vi "MainStateMachine.vi"() -> ()   [LabVIEW 2018]
uses:
  <vilib>/platform/TimedLoop/XDataNode/XDataNode.xnode
  <vilib>/Platform/TimedLoop/XDataNode/nitl_modes.ctl
  <vilib>/Platform/TimedLoop/XDataNode/XDNodeRunTimeDep.lvlib
  <vilib>/Platform/TimedLoop/XDataNode/wakeup.ctl
  <vilib>/Platform/TimedLoop/XDataNode/timing_clust.ctl
  Type_Def_ControlState.ctl
  <vilib>/Platform/TimedLoop/XDataNode/loadnilvce.vi
  Type_Def Actuator Controls.ctl
  C:/Users/eric/Documents/LabViewBuilds/Testing/FaultPractice/Type_Def SensorData.ctl
  2019_CompetitionCode-master/2019_CompetitionCode-master/Master/DAQ/TypeDef_cRIOData.ctl
panel:
  in  "error constant":errorcluster
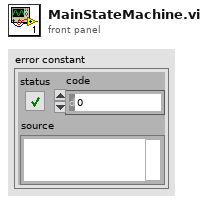
[diagram p1: front panel]
types:
  T1 = typedef "Type_Def Actuator Controls.ctl" = cluster{"Reverse ":bool, "Forward":bool, "Low Side":bool, "Precharge":bool, "High Side":bool, "Digital Out 5":bool, "Digital Out 6":bool, "Digital Out 7 ":bool, "24 Power":bool, "Tank Valve ":bool, "Brake Valve":bool, "Pump":bool, "Digital Out 1 ":bool, "Digital Out 2":bool, "Digital Out 3":bool, "Digital Out 4 ":bool}
  T2 = typedef "Type_Def_ControlState.ctl" = enum16{"Blank", "Systems Check", "Idle", "Ready", "Pushing", "CrawlingPrecharge", "Braking", "Fault", "Boot Up", "Unpowered", "Crawling", "Shutdown", "Service Push", "Service Wait", "Vent", "Precharge", "Cooldown"}
  T3 = typedef "Type_Def SensorData.ctl" = cluster{"cRIO Data":T4}
  T4 = typedef "TypeDef_cRIOData.ctl" = cluster{"Time (ms)":dbl, "24V Battery (V)":dbl, "LowV Current (A)":dbl, "Fiducial Sensor (V)":dbl, "PV Pressure (psig)":dbl, "Flow Sensor (V)":dbl, "Temp Fairing (F)":dbl, "Temp Reservoir (F)":dbl, "HallEffect Right (in)":dbl, "HallEffect Left (in)":dbl, "PT Tank (psig)":dbl, "PT Clamp Right (psig)":dbl, "PT Clamp Left (psig)":dbl, "PT Brake (psig)":dbl, "PT Cooling (psig)":dbl, "Displacement (ft)":dbl, "Velocity (ft/s)":dbl}
  T5 = cluster{"cRIO Data":cluster{"Time (ms)":dbl, "24V Battery (V)":dbl, "LowV Current (A)":dbl, "Fiducial Sensor (V)":dbl, "PV Pressure (psig)":dbl, "Flow Sensor (V)":dbl, "Temp Fairing (F)":dbl, "Temp Reservoir (F)":dbl, "HallEffect Right (in)":dbl, "HallEffect Left (in)":dbl, "PT Tank (psig)":dbl, "PT Clamp Right (psig)":dbl, "PT Clamp Left (psig)":dbl, "PT Brake (psig)":dbl, "PT Cooling (psig)":dbl, "Displacement (ft)":dbl, "Velocity (ft/s)":dbl}}
  T6 = typedef "Type_Def ClusterSensor.ctl" = cluster{"Sensor Data":dbl, "Max":dbl, "Min":dbl, "Previous Data":dbl, "#same":dbl}
  T7 = typedef "XDNodeRunTimeDep.lvlib/timing_clust.ctl" = cluster{"Expected End [f-1]":u64, "Actual End [f-1]":u64, "Finished Late? [f-1]":bool, "Expected End [i-1]":u64, "Actual End [i-1]":u64, "Finished Late? [i-1]":bool, "Expected Start [i]":u64, "Actual Start [i]":u64, "Expected Start [f]":u64, "Actual Start [f]":u64, "Source Name":string, "Structure Name":string, "Period":i64, "Deadline":i64, "Offset":i64, "Start":i64, "Priority":i32, "Timeout":i32, "Mode":T8, "Wakeup Reason":T9, "Error":errorcluster, "Source Type":string, "Secondary Source Type":string, "Global End Time":u64, "Global Start Time":u64, "Frame Duration":u64, "Iteration Duration":u64, "Assigned CPU":i32, "I/O Scan Engine Mode":u32}
  T8 = typedef "XDNodeRunTimeDep.lvlib/nitl_modes.ctl" = enum32{"No Change", "Process missed periods, maintain original phase", "Discard missed periods, maintain original phase", "Process missed periods, ignore original phase", "Discard missed periods, ignore original phase"}
  T9 = typedef "XDNodeRunTimeDep.lvlib/wakeup.ctl" = enum32{"Normal", "Aborted", "Asynchronous wakeup", "Timing source error", "Timed loop error", "Timeout"}
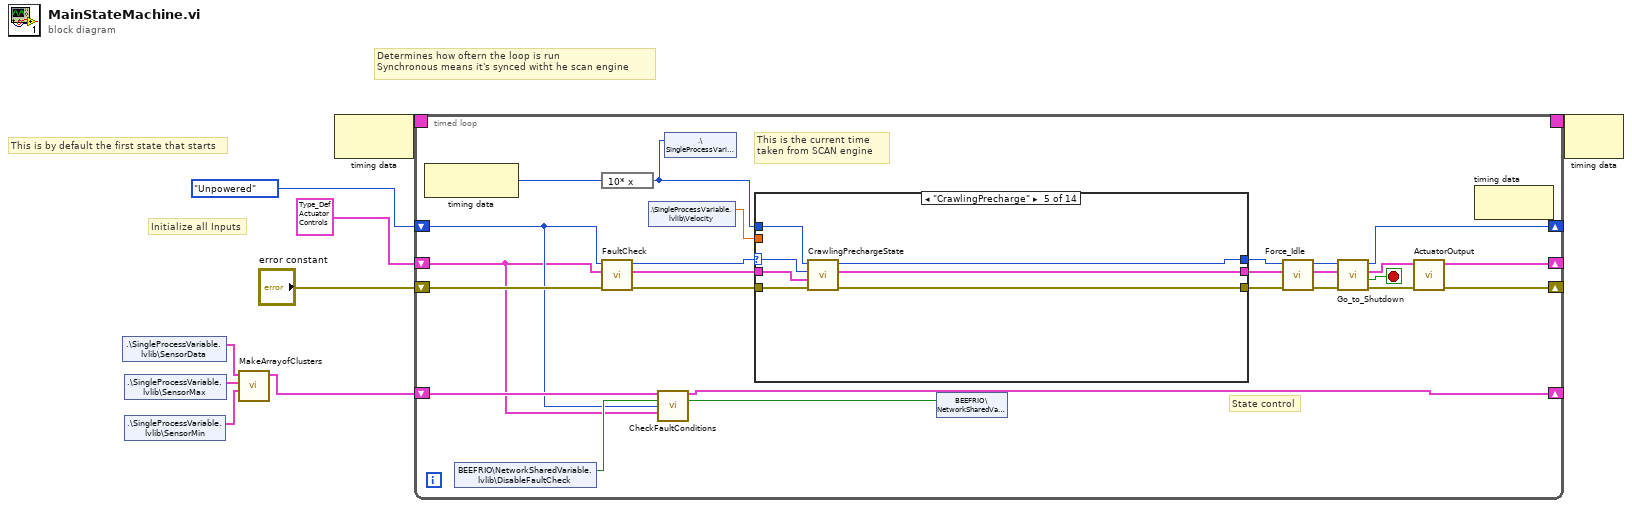
[diagram p0: block diagram]
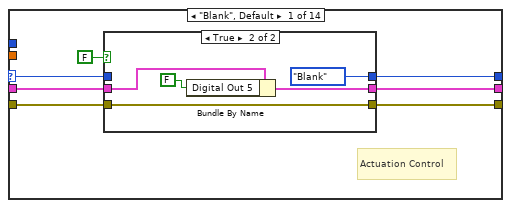
[diagram p2: hidden frame]
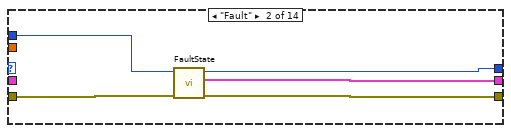
[diagram p4: hidden frame]
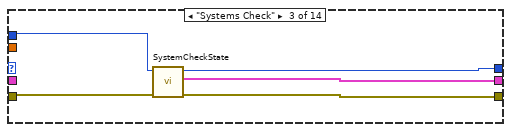
[diagram p5: hidden frame]
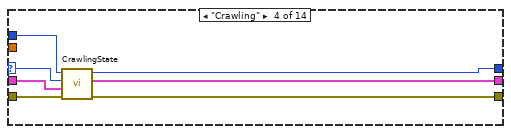
[diagram p6: hidden frame]
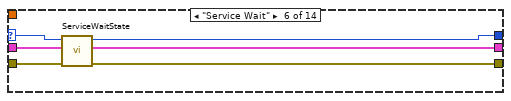
[diagram p7: hidden frame]
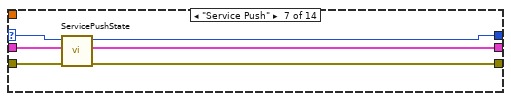
[diagram p8: hidden frame]
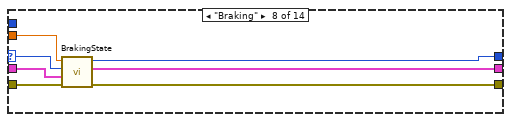
[diagram p9: hidden frame]
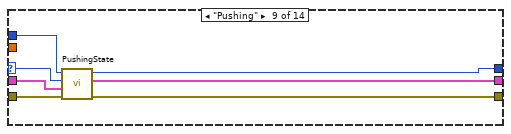
[diagram p10: hidden frame]
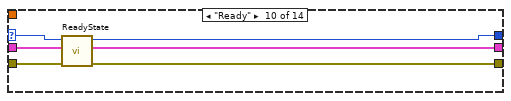
[diagram p11: hidden frame]
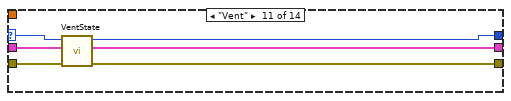
[diagram p12: hidden frame]
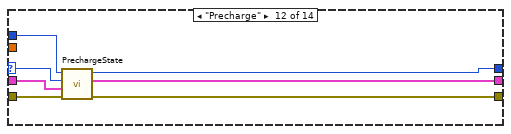
[diagram p13: hidden frame]
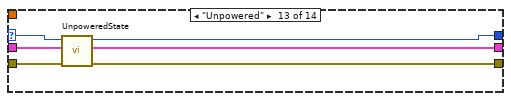
[diagram p14: hidden frame]
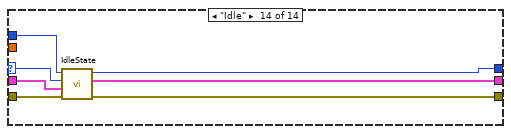
[diagram p15: hidden frame]
diagram:
  # "Determines how oftern the loop is run \nSynchronous means it's synced witht he scan engine"
  # "Initialize all Inputs"
  # "This is by default the first state that starts"
  n1 = shared-variable ".\\SingleProcessVariable.lvlib\\SensorData"() -> (w4:T3)  [unwired: 1 in, 1 out]
  n2 = shared-variable ".\\SingleProcessVariable.lvlib\\SensorMax"() -> (w3:T5)  [unwired: 1 in, 1 out]
  n3 = shared-variable ".\\SingleProcessVariable.lvlib\\SensorMin"() -> (w2:T3)  [unwired: 1 in, 1 out]
  n4 = call "MakeArrayofClusters.vi"(9:"SensorMax"=w2, 10:"SensorMax"=w3, "SensorData"=w4) -> ("Array"=w1:cluster{"SensorCluster":T6}[])  [unwired: 8 in]
  n5 = node-c288() -> (w9:T7)  [unwired: 1 in]
  n6 = timed-loop {
    timing: w9 -> [_]
    timing-out: [_] -> w8
    shift-right: [w33] -> _
    shift-left: Type_Def_ControlState."Unpowered" -> [w12]
    shift-right: [w21] -> _
    shift-left: T1 {"Reverse "=FALSE, "Forward"=FALSE, "Low Side"=FALSE, "Precharge"=FALSE, "High Side"=FALSE, "Digital Out 5"=FALSE, "Digital Out 6"=FALSE, "Digital Out 7 "=FALSE, "24 Power"=FALSE, "Tank Valve "=FALSE, "Brake Valve"=FALSE, "Pump"=FALSE, "Digital Out 1 "=FALSE, "Digital Out 2"=FALSE, "Digital Out 3"=FALSE, "Digital Out 4 "=FALSE} -> [w10]
    shift-right: [w20] -> _
    shift-left: "error constant" -> [w34]
    shift-right: [w15] -> _
    shift-left: w1 -> [w14]
    stop <- w24 stop-if-true
    # "This is the current time \ntaken from SCAN engine"
    # "State control"
    n7 = node-c288() -> (w23:i64)  [unwired: 1 in]
    n8 = shared-variable "BEEFRIO\\NetworkSharedVariable.lvlib\\DisableFaultCheck"() -> (w13:bool)  [unwired: 1 in, 1 out]
    n9 = expression code="10* x"(w23) -> (w22:i64)
    n10 = call "FaultCheck.vi"("error in (no error)"=w34, "Cluster in"=w10, "Enum in"=w12) -> ("error out"=w16:errorcluster, "Cluster out"=w17:T1, "Enum out"=w18:T2)  [unwired: 6 in]
    n11 = shared-variable ".\\SingleProcessVariable.lvlib\\Velocity"() -> (w19:dbl)  [unwired: 1 in, 1 out]
    n12 = call "CheckFaultConditions.vi"(0:w14, "DisableFaultCheck"=w13, "ControlState"=w12, "Cluster"=w10) -> ("Array out"=w15:cluster{"SensorCluster":T6}[], "Fault?"=w11:bool)  [unwired: 10 in]
    n13 = shared-variable ".\\SingleProcessVariable.lvlib\\Time"(w22) -> ()  [unwired: 1 in, 1 out]
    n14 = case shown="\"CrawlingPrecharge\"" w18 {
      selector: w18 -> [w41 _ _ w66 w73 w79 w85 w92 w99 w105 w111 w118 w124 w131]
      tunnel: [w40 w52 w57 w65 w72 w78 w84 w91 w98 w104 w110 w117 w123 w130] -> w28
      tunnel: [w38 w50 w55 w63 w70 w76 w82 w89 w96 w102 w108 w115 w121 w128] -> w31
      tunnel: w17 -> [w39 _ _ w64 w71 w77 w83 w90 w97 w103 w109 w116 w122 w129]
      tunnel: [w37 w51 w56 w62 w69 w75 w81 w88 w95 w101 w107 w114 w120 w127] -> w29
      tunnel: w16 -> [w36 w54 w58 w61 w68 w74 w80 w87 w94 w100 w106 w113 w119 w126]
      tunnel: w22 -> [_ w53 w59 w60 w67 _ _ _ w93 _ _ w112 _ w125]
      tunnel: w19 -> [_ _ _ _ _ _ _ w86 _ _ _ _ _ _]
      frame "Blank", Default {
        # "Actuation Control"
        n15 = case shown="True" FALSE {
          tunnel: w41 -> [w44 _]
          tunnel: [w44 Type_Def_ControlState."Blank"] -> w40
          tunnel: w39 -> [w43 w48]
          tunnel: [w43 w46] -> w38
          tunnel: [w42 w45] -> w37
          tunnel: w36 -> [w42 w45]
          frame False {
          }
          frame True {
            n16 = Bundle By Name(cluster=w48, "Digital Out 5"=FALSE) -> (w46:T1)
          }
        }
      }
      frame "Fault" {
        n17 = call "FaultState.vi"("error in (no error)"=w54, "Actual Start [i]"=w53) -> ("error out"=w51:errorcluster, "Cluster"=w50:T1, "Numeric"=w52:i64)  [unwired: 7 in]
      }
      frame "Systems Check" {
        n18 = call "SystemCheckState.vi"("error in (no error)"=w58, "Actual Start [i]"=w59) -> ("error out"=w56:errorcluster, "Cluster"=w55:T1, "Numeric"=w57:i64)  [unwired: 7 in]
      }
      frame "Crawling" {
        n19 = call "CrawlingState.vi"("error in (no error)"=w61, "Cluster in"=w64, "Enum in"=w66, "Actual Start [i]"=w60) -> ("error out"=w62:errorcluster, "Cluster out"=w63:T1, "Enum"=w65:T2)  [unwired: 5 in]
      }
      frame "CrawlingPrecharge" {
        n20 = call "CrawlingPrechargeState.vi"("error in (no error)"=w68, "Cluster in"=w71, "Enum in"=w73, "Actual Start [i]"=w67) -> ("error out"=w69:errorcluster, "Cluster out"=w70:T1, "Enum"=w72:T2)  [unwired: 5 in]
      }
      frame "Service Wait" {
        n21 = call "ServiceWaitState.vi"("error in (no error)"=w74, "Cluster in"=w77, "Enum in"=w79) -> ("error out"=w75:errorcluster, "Cluster out"=w76:T1, "Enum"=w78:T2)  [unwired: 6 in]
      }
      frame "Service Push" {
        n22 = call "ServicePushState.vi"("error in (no error)"=w80, "Cluster in"=w83, "Enum in"=w85) -> ("error out"=w81:errorcluster, "Cluster out"=w82:T1, "Enum out"=w84:T2)  [unwired: 6 in]
      }
      frame "Braking" {
        n23 = call "BrakingState.vi"("error in (no error)"=w87, "Cluster in"=w90, "Enum in"=w92, "Double"=w86) -> ("error out"=w88:errorcluster, "Cluster"=w89:T1, "Enum"=w91:T2)  [unwired: 5 in]
      }
      frame "Pushing" {
        n24 = call "PushingState.vi"("error in (no error)"=w94, "Cluster in"=w97, "Enum in"=w99, "Actual Start [i]"=w93) -> ("error out"=w95:errorcluster, "Cluster out"=w96:T1, "Enum"=w98:T2)  [unwired: 5 in]
      }
      frame "Ready" {
        n25 = call "ReadyState.vi"("error in (no error)"=w100, "Cluster in"=w103, "Enum in"=w105) -> ("error out"=w101:errorcluster, "Cluster out"=w102:T1, "Enum"=w104:T2)  [unwired: 6 in]
      }
      frame "Vent" {
        n26 = call "VentState.vi"("error in (no error)"=w106, "Cluster in"=w109, "Enum in"=w111) -> ("error out"=w107:errorcluster, "Cluster out"=w108:T1, "Enum out"=w110:T2)  [unwired: 6 in]
      }
      frame "Precharge" {
        n27 = call "PrechargeState.vi"("error in (no error)"=w113, "Cluster in"=w116, "Enum in"=w118, "Actual Start [i]"=w112) -> ("error out"=w114:errorcluster, "Cluster out"=w115:T1, "Enum"=w117:T2)  [unwired: 5 in]
      }
      frame "Unpowered" {
        n28 = call "UnpoweredState.vi"("error in (no error)"=w119, "Cluster in"=w122, "Enum in"=w124) -> ("error out"=w120:errorcluster, "Cluster out"=w121:T1, "Enum"=w123:T2)  [unwired: 6 in]
      }
      frame "Idle" {
        n29 = call "IdleState.vi"("error in (no error)"=w126, "Cluster in"=w129, "Enum in"=w131, "Actual Start [i]"=w125) -> ("error out"=w127:errorcluster, "Cluster out"=w128:T1, "Enum"=w130:T2)  [unwired: 5 in]
      }
    }
    n30 = shared-variable "BEEFRIO\\NetworkSharedVariable.lvlib\\Fault"(w11) -> ()  [unwired: 1 in, 1 out]
    n31 = call "Force_Idle.vi"("error in (no error)"=w29, "Cluster in"=w31, "Enum in"=w28) -> ("error out"=w26:errorcluster, "Cluster out"=w27:T1, "Enum out"=w25:T2)  [unwired: 6 in]
    n32 = call "Go_to_Shutdown.vi"("error in (no error)"=w26, "Cluster in"=w27, "Enum in"=w25) -> ("error out"=w30:errorcluster, "Stop State Machine"=w24:bool, "Cluster out"=w32:T1, "Enum out"=w33:T2)  [unwired: 5 in]
    n33 = call "ActuatorOutput.vi"("error in (no error)"=w30, "Cluster in"=w32) -> ("error out"=w20:errorcluster, "Cluster"=w21:T1)  [unwired: 8 in]
    n34 = node-c288() -> ()  [unwired: 1 in, 1 out]
  }
  n35 = node-c288(w8) -> ()  [unwired: 1 out]
